vi "read_IMU Main_simple_Robot.vi"(8 "error in (no error)":errorcluster) -> (0 "error out":errorcluster)   [LabVIEW 2013]
uses:
  IMU_Data_Type_Def.ctl
  My Computer/Controls/Sensors State.ctl
panel:
  out "IMU_Data_simple":T1
  out "Elapsed Loop time [ms]":u32
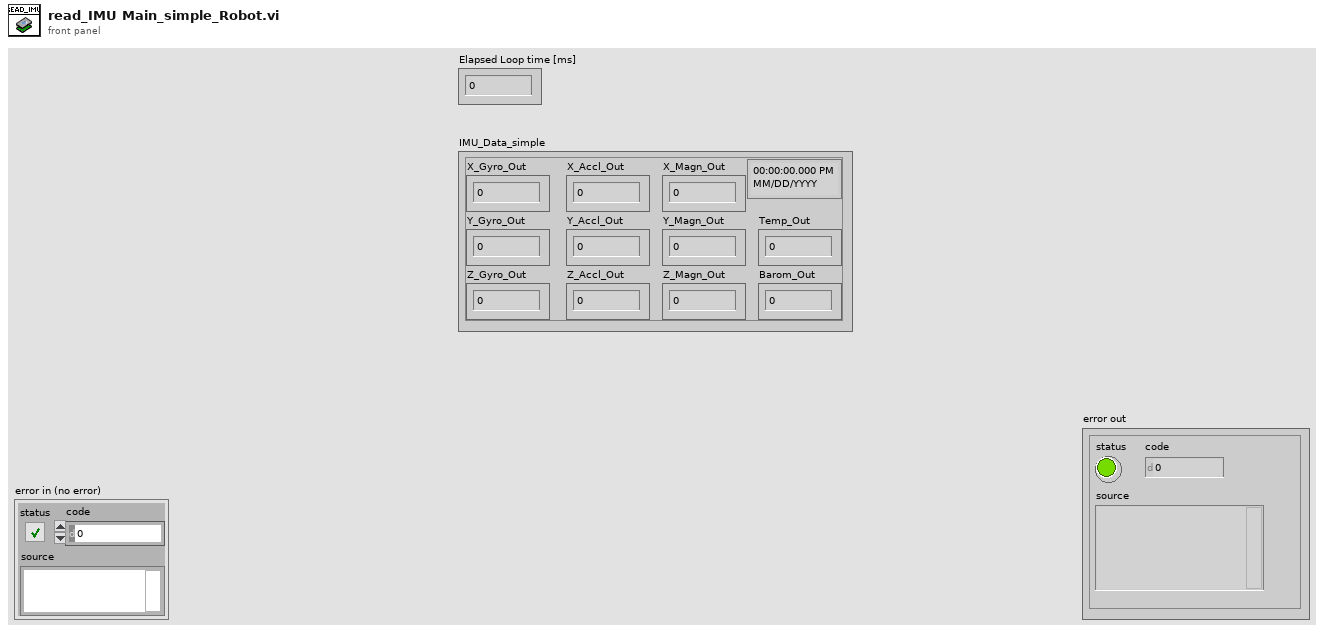
[diagram p1: front panel]
types:
  T1 = typedef "IMU_Data_Type_Def.ctl" = cluster{timestamp, "X_Gyro_Out":dbl, "Y_Gyro_Out":dbl, "Z_Gyro_Out":dbl, "X_Accl_Out":dbl, "Y_Accl_Out":dbl, "Z_Accl_Out":dbl, "X_Magn_Out":dbl, "Y_Magn_Out":dbl, "Z_Magn_Out":dbl, "Temp_Out":dbl, "Barom_Out":dbl}
  T2 = typedef "Sensors State.ctl" = cluster{"Leakage-Sensor_enabled":bool, "IMU_enabled":bool, "Swimbladder Fill-State-Sensor_enabled":bool, "Flow-Sensor_enabled":bool, "Depth-Sensor_enabled":bool, "Current-Sensor_enabled":bool, "Calibrate Depth":bool, "SB_Piston_Stuck_Detect_enabled":bool, "Check_too_Deep_enabled":bool}
  T3 = cluster{timestamp, "Scaled Measurement 1":dbl, "Scaled last Measurement":dbl, "Scaled Measurement 1":dbl, "Scaled last Measurement":dbl, "Scaled Measurement 1":dbl, "Scaled last Measurement":dbl, "Scaled Measurement 1":dbl, "Scaled last Measurement":dbl, "Scaled Measurement 1":dbl, "Scaled last Measurement":dbl, "Scaled Measurement 1":dbl}
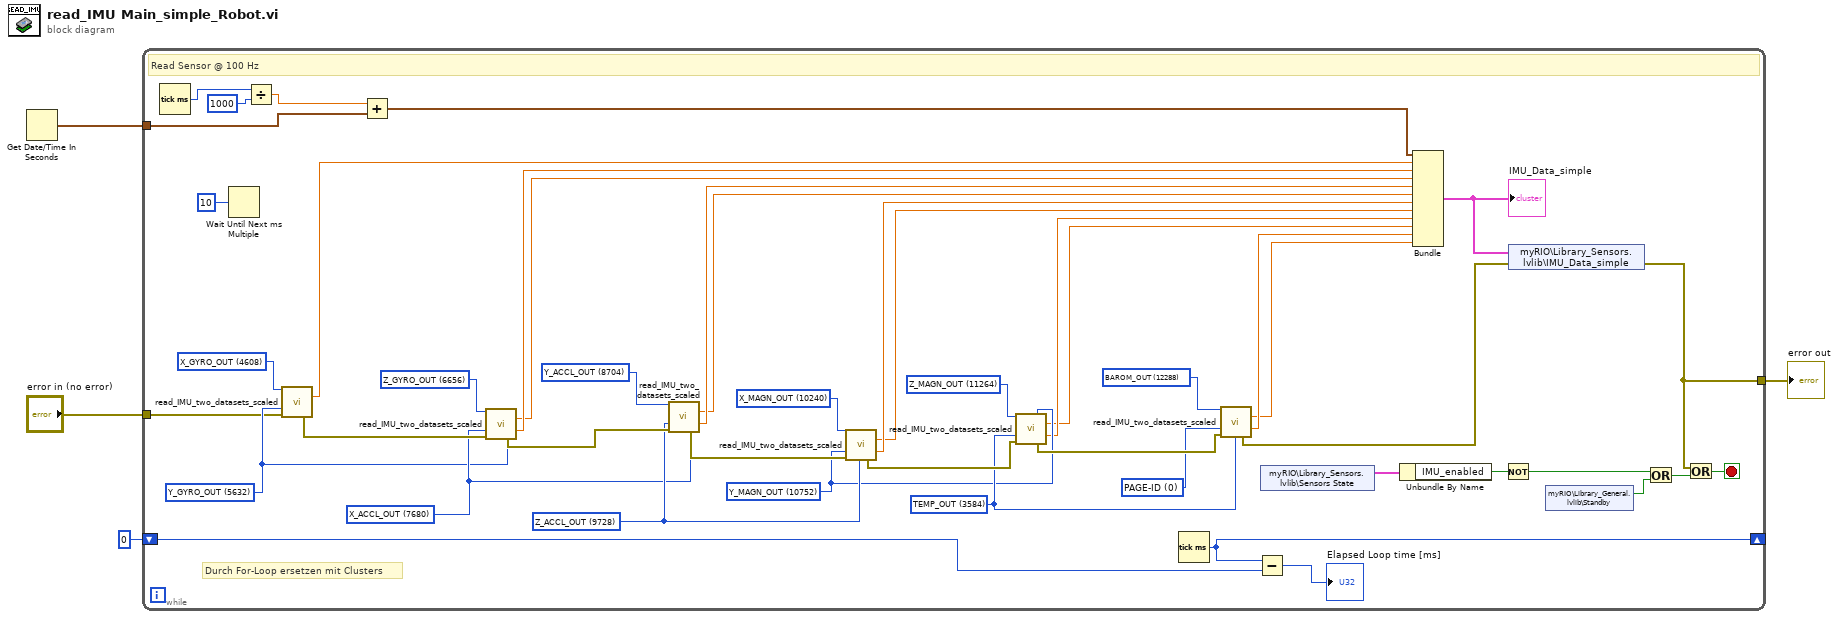
[diagram p0: block diagram]
diagram:
  n1 = Get Date/Time In Seconds() -> (seconds since 1Jan1904=w4:timestamp)
  n2 = while {
    shift-right: [w37] -> _
    shift-left: u32 0 ("millisecond timer value") -> [w38]
    tunnel: w4 -> [w34]
    tunnel: [w11] -> w2
    tunnel: "error in (no error)" -> [w6]
    stop <- w39 stop-if-true
    w33 = u16 0 items=["PAGE-ID"=0, "SYS_E_FLAG"=2048, "DIAG_STS"=2560, "ALM_STS"=3072, "TEMP_OUT"=3584, "X_GYRO_OUT"=4608, "Y_GYRO_OUT"=5632, "Z_GYRO_OUT"=6656, "X_ACCL_OUT"=7680, "Y_ACCL_OUT"=8704, "Z_ACCL_OUT"=9728, "X_MAGN_OUT"=10240, "Y_MAGN_OUT"=10752, "Z_MAGN_OUT"=11264, "BAROM_OUT"=12288, "X_DELTAANG_OUT"=16896, "Y_DELTAANG_OUT"=17920, "Z_DELTAANG_OUT"=18944, "X_DELTAVEL_OUT"=19968, "Y_DELTAVEL_OUT"=20992, "Z_DELTAVEL_OUT"=22016] ("Measurement Type 1")
    w45 = u16 12288 items=["PAGE-ID"=0, "SYS_E_FLAG"=2048, "DIAG_STS"=2560, "ALM_STS"=3072, "TEMP_OUT"=3584, "X_GYRO_OUT"=4608, "Y_GYRO_OUT"=5632, "Z_GYRO_OUT"=6656, "X_ACCL_OUT"=7680, "Y_ACCL_OUT"=8704, "Z_ACCL_OUT"=9728, "X_MAGN_OUT"=10240, "Y_MAGN_OUT"=10752, "Z_MAGN_OUT"=11264, "BAROM_OUT"=12288, "X_DELTAANG_OUT"=16896, "Y_DELTAANG_OUT"=17920, "Z_DELTAANG_OUT"=18944, "X_DELTAVEL_OUT"=19968, "Y_DELTAVEL_OUT"=20992, "Z_DELTAVEL_OUT"=22016] ("Measurement Type 1")
    w35 = u16 3584 items=["PAGE-ID"=0, "SYS_E_FLAG"=2048, "DIAG_STS"=2560, "ALM_STS"=3072, "TEMP_OUT"=3584, "X_GYRO_OUT"=4608, "Y_GYRO_OUT"=5632, "Z_GYRO_OUT"=6656, "X_ACCL_OUT"=7680, "Y_ACCL_OUT"=8704, "Z_ACCL_OUT"=9728, "X_MAGN_OUT"=10240, "Y_MAGN_OUT"=10752, "Z_MAGN_OUT"=11264, "BAROM_OUT"=12288, "X_DELTAANG_OUT"=16896, "Y_DELTAANG_OUT"=17920, "Z_DELTAANG_OUT"=18944, "X_DELTAVEL_OUT"=19968, "Y_DELTAVEL_OUT"=20992, "Z_DELTAVEL_OUT"=22016] ("Measurement Type 2")
    w46 = u16 11264 items=["PAGE-ID"=0, "SYS_E_FLAG"=2048, "DIAG_STS"=2560, "ALM_STS"=3072, "TEMP_OUT"=3584, "X_GYRO_OUT"=4608, "Y_GYRO_OUT"=5632, "Z_GYRO_OUT"=6656, "X_ACCL_OUT"=7680, "Y_ACCL_OUT"=8704, "Z_ACCL_OUT"=9728, "X_MAGN_OUT"=10240, "Y_MAGN_OUT"=10752, "Z_MAGN_OUT"=11264, "BAROM_OUT"=12288, "X_DELTAANG_OUT"=16896, "Y_DELTAANG_OUT"=17920, "Z_DELTAANG_OUT"=18944, "X_DELTAVEL_OUT"=19968, "Y_DELTAVEL_OUT"=20992, "Z_DELTAVEL_OUT"=22016] ("Measurement Type 1")
    w29 = u16 10752 items=["PAGE-ID"=0, "SYS_E_FLAG"=2048, "DIAG_STS"=2560, "ALM_STS"=3072, "TEMP_OUT"=3584, "X_GYRO_OUT"=4608, "Y_GYRO_OUT"=5632, "Z_GYRO_OUT"=6656, "X_ACCL_OUT"=7680, "Y_ACCL_OUT"=8704, "Z_ACCL_OUT"=9728, "X_MAGN_OUT"=10240, "Y_MAGN_OUT"=10752, "Z_MAGN_OUT"=11264, "BAROM_OUT"=12288, "X_DELTAANG_OUT"=16896, "Y_DELTAANG_OUT"=17920, "Z_DELTAANG_OUT"=18944, "X_DELTAVEL_OUT"=19968, "Y_DELTAVEL_OUT"=20992, "Z_DELTAVEL_OUT"=22016] ("Measurement Type 2")
    w47 = u16 10240 items=["PAGE-ID"=0, "SYS_E_FLAG"=2048, "DIAG_STS"=2560, "ALM_STS"=3072, "TEMP_OUT"=3584, "X_GYRO_OUT"=4608, "Y_GYRO_OUT"=5632, "Z_GYRO_OUT"=6656, "X_ACCL_OUT"=7680, "Y_ACCL_OUT"=8704, "Z_ACCL_OUT"=9728, "X_MAGN_OUT"=10240, "Y_MAGN_OUT"=10752, "Z_MAGN_OUT"=11264, "BAROM_OUT"=12288, "X_DELTAANG_OUT"=16896, "Y_DELTAANG_OUT"=17920, "Z_DELTAANG_OUT"=18944, "X_DELTAVEL_OUT"=19968, "Y_DELTAVEL_OUT"=20992, "Z_DELTAVEL_OUT"=22016] ("Measurement Type 1")
    w32 = u16 9728 items=["PAGE-ID"=0, "SYS_E_FLAG"=2048, "DIAG_STS"=2560, "ALM_STS"=3072, "TEMP_OUT"=3584, "X_GYRO_OUT"=4608, "Y_GYRO_OUT"=5632, "Z_GYRO_OUT"=6656, "X_ACCL_OUT"=7680, "Y_ACCL_OUT"=8704, "Z_ACCL_OUT"=9728, "X_MAGN_OUT"=10240, "Y_MAGN_OUT"=10752, "Z_MAGN_OUT"=11264, "BAROM_OUT"=12288, "X_DELTAANG_OUT"=16896, "Y_DELTAANG_OUT"=17920, "Z_DELTAANG_OUT"=18944, "X_DELTAVEL_OUT"=19968, "Y_DELTAVEL_OUT"=20992, "Z_DELTAVEL_OUT"=22016] ("Measurement Type 2")
    w49 = u16 8704 items=["PAGE-ID"=0, "SYS_E_FLAG"=2048, "DIAG_STS"=2560, "ALM_STS"=3072, "TEMP_OUT"=3584, "X_GYRO_OUT"=4608, "Y_GYRO_OUT"=5632, "Z_GYRO_OUT"=6656, "X_ACCL_OUT"=7680, "Y_ACCL_OUT"=8704, "Z_ACCL_OUT"=9728, "X_MAGN_OUT"=10240, "Y_MAGN_OUT"=10752, "Z_MAGN_OUT"=11264, "BAROM_OUT"=12288, "X_DELTAANG_OUT"=16896, "Y_DELTAANG_OUT"=17920, "Z_DELTAANG_OUT"=18944, "X_DELTAVEL_OUT"=19968, "Y_DELTAVEL_OUT"=20992, "Z_DELTAVEL_OUT"=22016] ("Measurement Type 1")
    w31 = u16 7680 items=["PAGE-ID"=0, "SYS_E_FLAG"=2048, "DIAG_STS"=2560, "ALM_STS"=3072, "TEMP_OUT"=3584, "X_GYRO_OUT"=4608, "Y_GYRO_OUT"=5632, "Z_GYRO_OUT"=6656, "X_ACCL_OUT"=7680, "Y_ACCL_OUT"=8704, "Z_ACCL_OUT"=9728, "X_MAGN_OUT"=10240, "Y_MAGN_OUT"=10752, "Z_MAGN_OUT"=11264, "BAROM_OUT"=12288, "X_DELTAANG_OUT"=16896, "Y_DELTAANG_OUT"=17920, "Z_DELTAANG_OUT"=18944, "X_DELTAVEL_OUT"=19968, "Y_DELTAVEL_OUT"=20992, "Z_DELTAVEL_OUT"=22016] ("Measurement Type 2")
    w50 = u16 6656 items=["PAGE-ID"=0, "SYS_E_FLAG"=2048, "DIAG_STS"=2560, "ALM_STS"=3072, "TEMP_OUT"=3584, "X_GYRO_OUT"=4608, "Y_GYRO_OUT"=5632, "Z_GYRO_OUT"=6656, "X_ACCL_OUT"=7680, "Y_ACCL_OUT"=8704, "Z_ACCL_OUT"=9728, "X_MAGN_OUT"=10240, "Y_MAGN_OUT"=10752, "Z_MAGN_OUT"=11264, "BAROM_OUT"=12288, "X_DELTAANG_OUT"=16896, "Y_DELTAANG_OUT"=17920, "Z_DELTAANG_OUT"=18944, "X_DELTAVEL_OUT"=19968, "Y_DELTAVEL_OUT"=20992, "Z_DELTAVEL_OUT"=22016] ("Measurement Type 1")
    w30 = u16 5632 items=["PAGE-ID"=0, "SYS_E_FLAG"=2048, "DIAG_STS"=2560, "ALM_STS"=3072, "TEMP_OUT"=3584, "X_GYRO_OUT"=4608, "Y_GYRO_OUT"=5632, "Z_GYRO_OUT"=6656, "X_ACCL_OUT"=7680, "Y_ACCL_OUT"=8704, "Z_ACCL_OUT"=9728, "X_MAGN_OUT"=10240, "Y_MAGN_OUT"=10752, "Z_MAGN_OUT"=11264, "BAROM_OUT"=12288, "X_DELTAANG_OUT"=16896, "Y_DELTAANG_OUT"=17920, "Z_DELTAANG_OUT"=18944, "X_DELTAVEL_OUT"=19968, "Y_DELTAVEL_OUT"=20992, "Z_DELTAVEL_OUT"=22016] ("Measurement Type 2")
    w41 = u16 4608 items=["PAGE-ID"=0, "SYS_E_FLAG"=2048, "DIAG_STS"=2560, "ALM_STS"=3072, "TEMP_OUT"=3584, "X_GYRO_OUT"=4608, "Y_GYRO_OUT"=5632, "Z_GYRO_OUT"=6656, "X_ACCL_OUT"=7680, "Y_ACCL_OUT"=8704, "Z_ACCL_OUT"=9728, "X_MAGN_OUT"=10240, "Y_MAGN_OUT"=10752, "Z_MAGN_OUT"=11264, "BAROM_OUT"=12288, "X_DELTAANG_OUT"=16896, "Y_DELTAANG_OUT"=17920, "Z_DELTAANG_OUT"=18944, "X_DELTAVEL_OUT"=19968, "Y_DELTAVEL_OUT"=20992, "Z_DELTAVEL_OUT"=22016] ("Measurement Type 1")
    # "Durch For-Loop ersetzen mit Clusters"
    # "Read Sensor @ 100 Hz"
    n3 = Tick Count (ms)() -> (millisecond timer value=w15:u32)
    n4 = Wait Until Next ms Multiple(millisecond multiple=u32 10 ("milliseconds to wait")) -> ()  [unwired: 1 out]
    n5 = Divide(x=w15, y=u32 1000) -> (x/y=w13:dbl)
    n6 = call "read_IMU_two_datasets_scaled.vi"("First Measurement Type"=w41, "Next Measurement Type"=w30, "error in (no error)"=w6) -> ("Scaled Measurement 1"=w28:dbl, "error out"=w40:errorcluster)  [unwired: 6 in, 5 out]
    n7 = Add(x=w13, y=w34) -> (x+y=w17:timestamp)
    n8 = call "read_IMU_two_datasets_scaled.vi"("First Measurement Type"=w50, "Last Measurement Type"=w30, "Next Measurement Type"=w31, "error in (no error)"=w40) -> ("Scaled Measurement 1"=w26:dbl, "Scaled last Measurement"=w27:dbl, "error out"=w48:errorcluster)  [unwired: 5 in, 4 out]
    n9 = call "read_IMU_two_datasets_scaled.vi"("First Measurement Type"=w49, "Last Measurement Type"=w31, "Next Measurement Type"=w32, "error in (no error)"=w48) -> ("Scaled Measurement 1"=w24:dbl, "Scaled last Measurement"=w25:dbl, "error out"=w44:errorcluster)  [unwired: 5 in, 4 out]
    n10 = call "read_IMU_two_datasets_scaled.vi"("First Measurement Type"=w47, "Last Measurement Type"=w32, "Next Measurement Type"=w29, "error in (no error)"=w44) -> ("Scaled Measurement 1"=w22:dbl, "Scaled last Measurement"=w23:dbl, "error out"=w43:errorcluster)  [unwired: 5 in, 4 out]
    n11 = call "read_IMU_two_datasets_scaled.vi"("First Measurement Type"=w46, "Last Measurement Type"=w29, "Next Measurement Type"=w35, "error in (no error)"=w43) -> ("Scaled Measurement 1"=w20:dbl, "Scaled last Measurement"=w21:dbl, "error out"=w42:errorcluster)  [unwired: 5 in, 4 out]
    n12 = Tick Count (ms)() -> (millisecond timer value=w37:u32)
    n13 = call "read_IMU_two_datasets_scaled.vi"("First Measurement Type"=w45, "Last Measurement Type"=w35, "Next Measurement Type"=w33, "error in (no error)"=w42) -> ("Scaled Measurement 1"=w18:dbl, "Scaled last Measurement"=w19:dbl, "error out"=w12:errorcluster)  [unwired: 5 in, 4 out]
    n14 = Subtract(x=w37, y=w38) -> (x-y=→"Elapsed Loop time [ms]":u32)
    n15 = shared-variable "myRIO\\Library_Sensors.lvlib\\Sensors State"() -> (w10:T2)  [unwired: 1 in, 1 out]
    n16 = Unbundle By Name(w10) -> ("IMU_enabled"=w5:bool)
    n17 = Bundle(w17, "Scaled Measurement 1"=w28, "Scaled last Measurement"=w27, "Scaled Measurement 1"=w26, "Scaled last Measurement"=w25, "Scaled Measurement 1"=w24, "Scaled last Measurement"=w23, "Scaled Measurement 1"=w22, "Scaled last Measurement"=w21, "Scaled Measurement 1"=w20, "Scaled last Measurement"=w19, "Scaled Measurement 1"=w18) -> (w16:T3)  [unwired: 1 in]
    "IMU_Data_simple" <- w16
    n18 = Not(x=w5) -> (.not. x?=w9:bool)
    n19 = shared-variable "myRIO\\Library_Sensors.lvlib\\IMU_Data_simple"(w16, error in=w12) -> (error out=w11:errorcluster)
    n20 = shared-variable "myRIO\\Library_General.lvlib\\Standby"() -> (w8:bool)  [unwired: 1 in, 1 out]
    n21 = Or(x=w9, y=w8) -> (x .or. y?=w7:bool)
    n22 = Or(x=w11, y=w7) -> (x .or. y?=w39:bool)
  }
  "error out" <- w2
